vi "2 memory dds 8SPC.vi"(8 "referenses":T1={"clock x2"="IO Socket\\Data Clock 2x", "Memory In"="pulse on memory", "Memory In 2"="pulse on memory"}, 9 "pdw in":T3 {"frequency shift" format="%#_12f"}, 10 "free DDS before me?":bool, 11 "new PDW in":bool) -> (0 "output valid":bool, 1 "state of every DDS":bool[](array[boolean]), 2 "have free DDS":bool, 3 "IQ out":T2[](array[typedef]))   [LabVIEW 2021]
doc: "transmit pulse with one free DDS inside.\nmust have no DDS before him (the distribute is to give the lowest mun DDS the pulse)"
uses:
  pulse_tx_vis/pdw.ctl
  pulse_tx_vis/CTL/mode_type.ctl
  <instrlib>/_niInstr/DSP/v1/Shared/Public/IQ Data.ctl
  <instrlib>/_niInstr/DSP/v1/Shared/niInstr DSP v1 Shared.lvlib
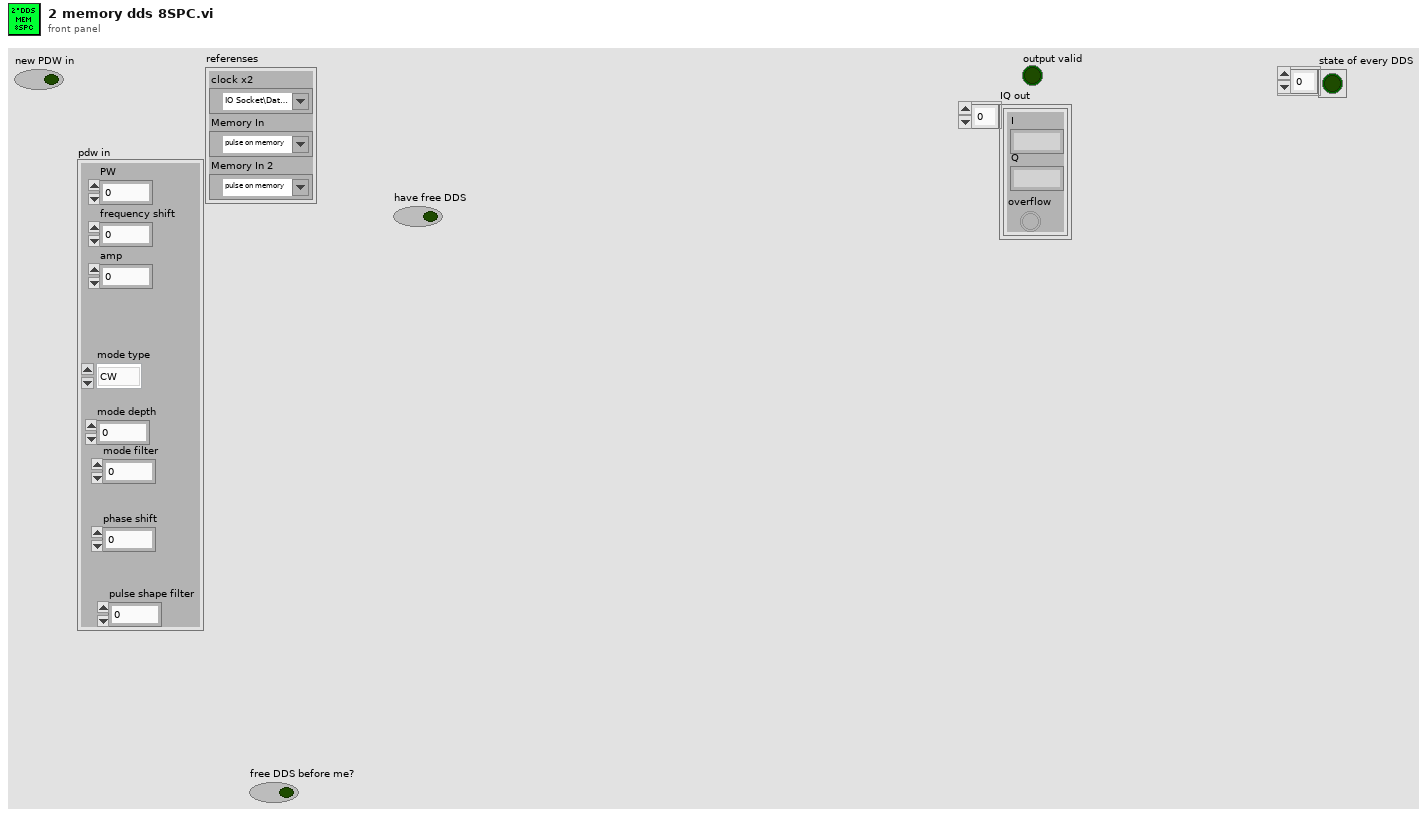
[diagram p1: front panel]
types:
  T1 = cluster{"clock x2":refnum<k21>, "Memory In":refnum<k21>, "Memory In 2":refnum<k21>}
  T2 = typedef "niInstr DSP v1 Shared.lvlib/IQ Data.ctl" = cluster{"I":fxp<+/-,18,1>, "Q":fxp<+/-,18,1>, "overflow":bool}
  T3 = typedef "pdw.ctl" = cluster{"PW":u32, "frequency shift":fxp<+/-,48,0>, "amp":fxp<+/-,18,1>, "mode type":T4, "mode depth":u32, "mode filter":u8, "phase shift":fxp<+/-,16,1>, "pulse shape filter":u8}
  T4 = typedef "mode_type.ctl" = enum8{"CW", "from memory 1", "NC - cw", "LFM", "BPSK", "QPSK"}
  T5 = cluster{"clock x2":refnum<k21>, "Memory In":refnum<k21>}
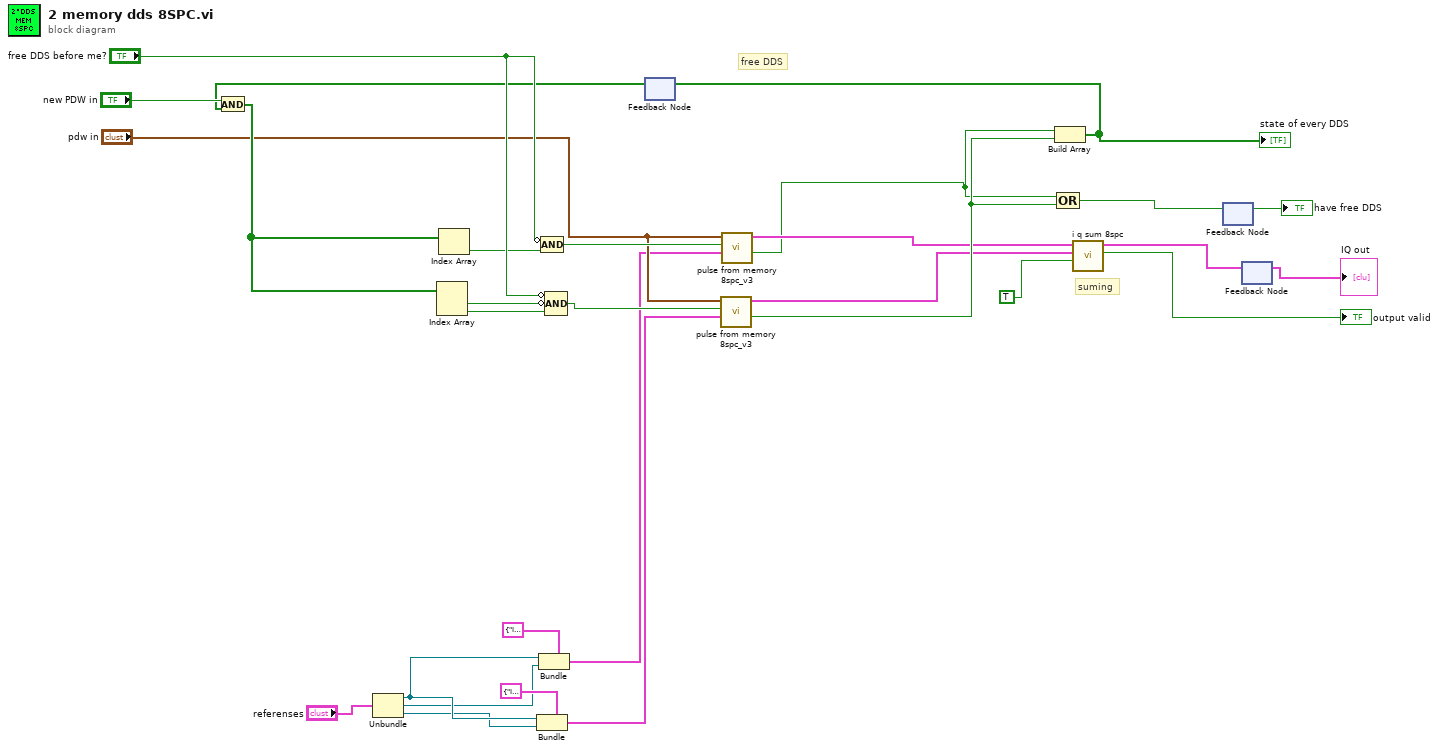
[diagram p0: block diagram]
diagram:
  # "free DDS"
  # "suming"
  n1 = Unbundle("referenses") -> ("clock x2"=w6:refnum<k21>, "Memory In"=w4:refnum<k21>, "Memory In 2"=w5:refnum<k21>)
  n2 = Bundle(cluster=T5 {"clock x2"="IO Socket\\Data Clock 2x", "Memory In"="pulse on memory"} ("referenses"), "clock x2"=w6, "Memory In"=w5) -> (w2:T5)
  n3 = Bundle(cluster=T5 {"clock x2"="IO Socket\\Data Clock 2x", "Memory In"="pulse on memory"} ("referenses"), "clock x2"=w6, "Memory In"=w4) -> (w3:T5)
  n4 = feedback #1() -> (w18:bool[])  [unwired: 1 in]
  n5 = And(x="new PDW in", y=w18) -> (x .and. y?=w17:bool[])
  n6 = Index Array(array=w17) -> (element #1=w27:bool, element #2=w25:bool)  [unwired: 2 in]
  n7 = Index Array(array=w17) -> (element=w23:bool)  [unwired: 1 in]
  n8 = Compound Arithmetic op=AND(invert "free DDS before me?", w23) -> (w24:bool)
  n9 = Compound Arithmetic op=AND(invert "free DDS before me?", invert w27, w25) -> (w26:bool)
  n10 = call "pulse from memory 8spc_v3.vi"("referenses"=w2, "start this pulse"=w26, "PDW"="pdw in") -> ("free DDS"=w28:bool, "IQ_out"=w22:T2[])  [unwired: 7 in]
  n11 = call "pulse from memory 8spc_v3.vi"("referenses"=w3, "start this pulse"=w24, "PDW"="pdw in") -> ("free DDS"=w11:bool, "IQ_out"=w21:T2[])  [unwired: 7 in]
  n12 = Build Array(w11, w28) -> (w20:bool[])
  "state of every DDS" <- w20
  n13 = feedback-in #1(w20) -> ()
  n14 = Compound Arithmetic op=OR(w11, w28) -> (w16:bool)
  n15 = call "i q sum 8spc.vi"("input valid"=TRUE, "IQ in 2"=w22, "IQ in"=w21) -> ("output valid"=→"output valid":bool, "IQ out"=w13:T2[])  [unwired: 7 in]
  n16 = feedback #2() -> (→"have free DDS":bool)  [unwired: 1 in]
  n17 = feedback-in #2(w16) -> ()
  n18 = feedback #3() -> (→"IQ out":T2[])  [unwired: 1 in]
  n19 = feedback-in #3(w13) -> ()
